vi "Destroy Client.vi"(8 "error in":errorcluster) -> (0 "error out":errorcluster)   [LabVIEW 2021, in "NI Pin Map V1 Client.lvlib"]
uses:
  NI Pin Map V1 Client.lvlib
  Discovery V1/TypeDefs/gRPC Client Cache FGV Action.ctl
  Discovery V1/NI Discovery V1 Client.lvlib
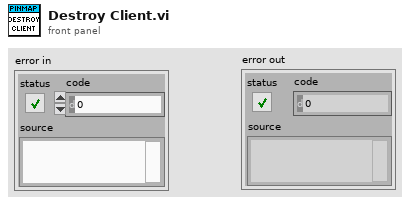
[diagram p1: front panel]
types:
  T1 = typedef "NI Discovery V1 Client.lvlib/gRPC Client Cache FGV Action.ctl" = enum16{"Get Client", "Recreate Client", "Destroy Client", "Update ClusterId"}
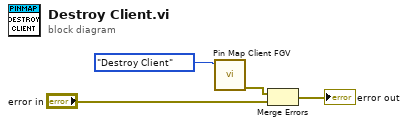
[diagram p0: block diagram]
diagram:
  n1 = call "Pin Map Client FGV.vi"("action"=gRPC_Client_Cache_FGV_Action."Destroy Client") -> ("error out"=w1:errorcluster)  [unwired: 8 in, 2 out]
  n2 = Merge Errors(w1, "error in") -> (→"error out":errorcluster)
